vi "Setup.vi"() -> ()   [LabVIEW 2014]
uses:
  Controls/State typedef.ctl
  <vilib>/vision/NI_Vision_Development_Module.lvlib
panel:
  in  "update":bool
  out "updating":i32(slide)=250 scale=0.0..250.0
  in  "Progress...":u32(slide) min=400 max=47374 scale=0.0..21744.0
  in  "hori":cluster{i32, i32}(slide) scale=0.0..720.0
  in  "vert":cluster{i32, i32}(slide)
  out "Video play":T1(plugin-control)
  in  "START":bool
  in  "Data file":path caption="Data"
  in  "Video file":path caption="Video"
  in  "Set end":bool
  out "Start":dbl=1.0 min=0.25 max=4.0 step=0.25
  in  "Set start":bool
  out "End":dbl=1.0 min=0.25 max=4.0 step=0.25
  in  "Pause Button 2":bool
  in  "Play back\nsettings":dbl=1.0 min=0.25 max=4.0 step=0.25
  out "output array":dbl[](array[numeric])
  in  "frame jump":i32=1 min=1 max=30
  in  "Seek Forward Button":bool
  in  "Seek Back Button":bool
  in  "Pause Button":bool
  in  "Media Stop Button":bool
  in  "Play Button":bool
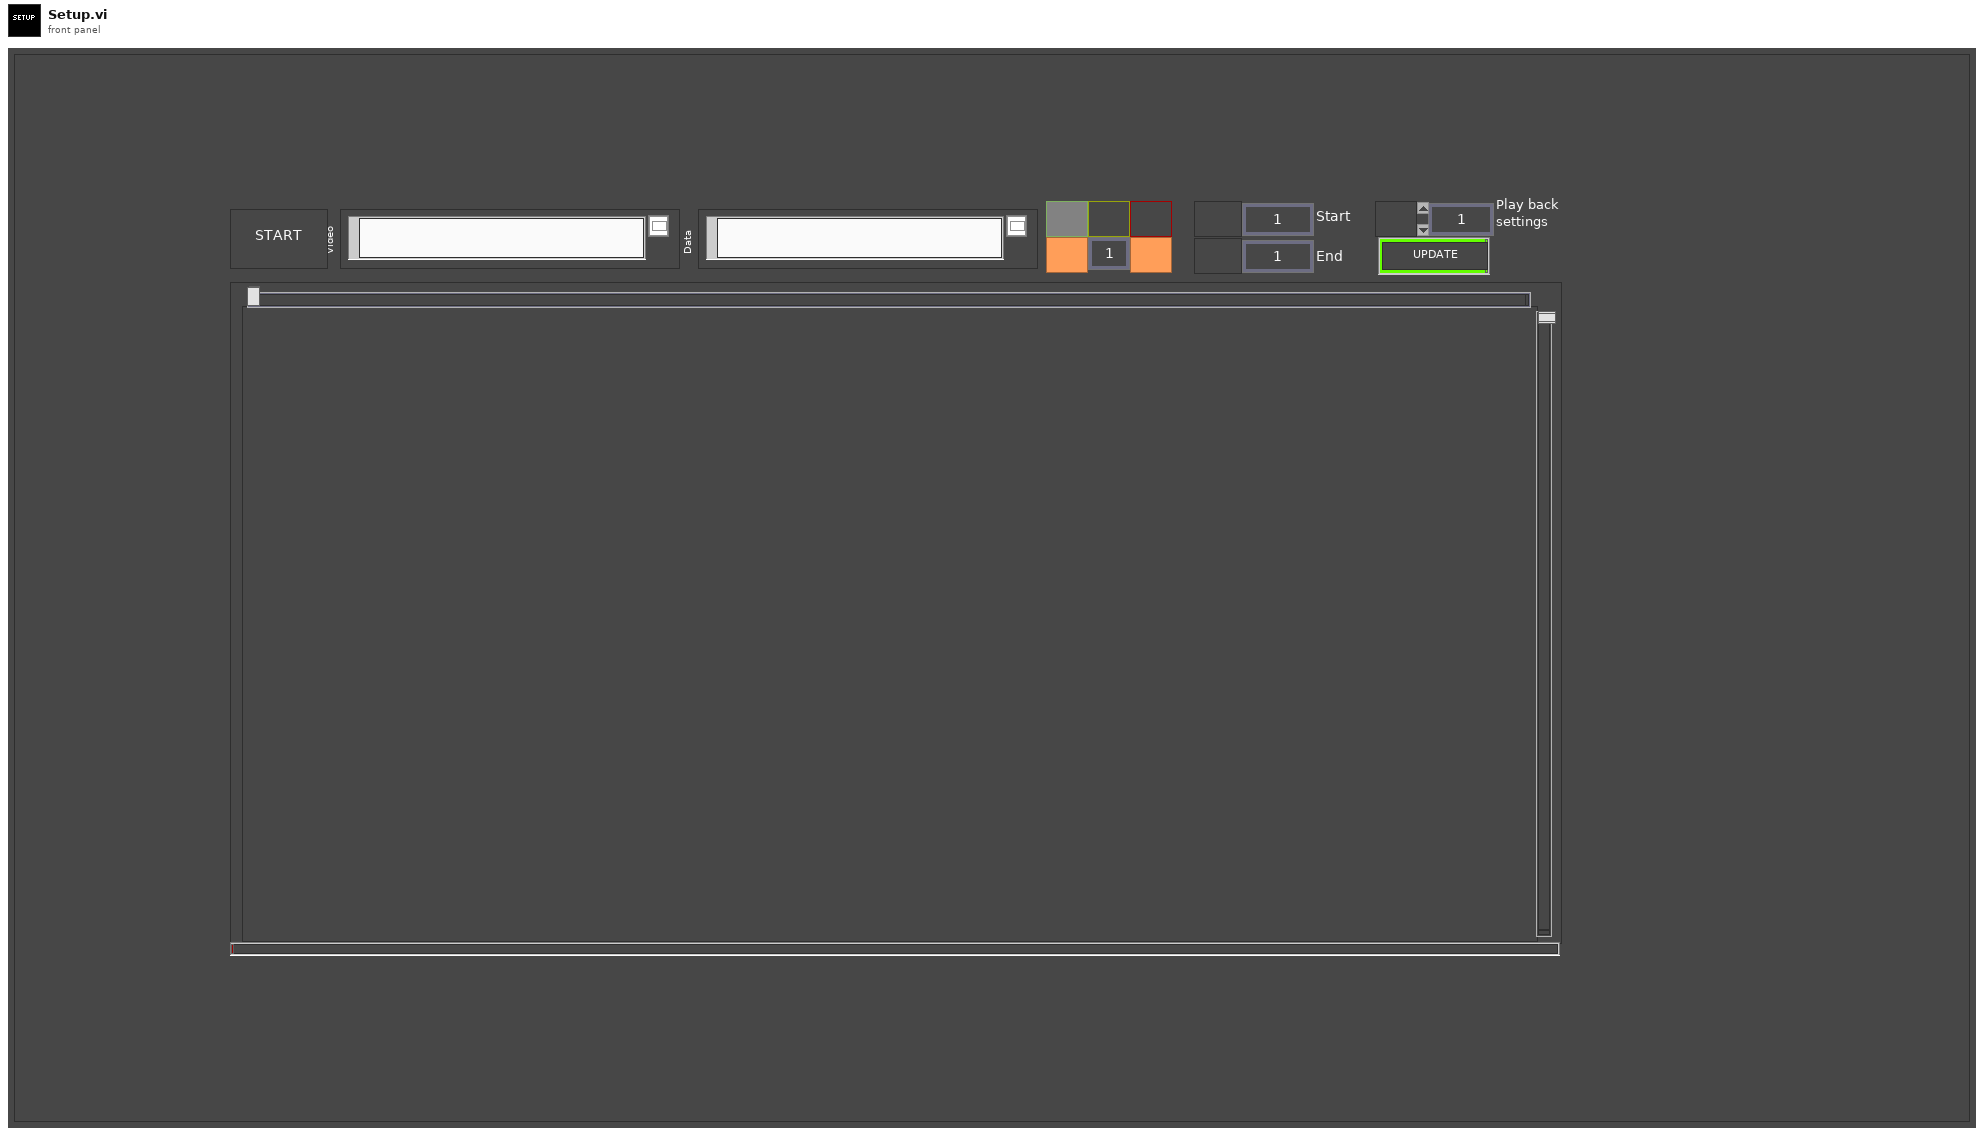
[diagram p1: front panel]
types:
  T1 = typedef "IMAQ Image.ctl" = refnum<image>
  T2 = typedef "State typedef.ctl" = enum16{"innit", "stop", "Pause", "Play", "Wait", "update"}
  T3 = typedef "Image Type" = u32
  T4 = enum16{"open", "replace", "create", "open or create", "replace or create", "replace or create with confirmation"}
  T5 = typedef "AviRefnum.ctl" = refnum<k1>
  T6 = cluster{"width":u32, "height":u32, "framesPerSecond":u32, "compressionFilter":string, "hasData":bool}
  T7 = cluster{"ID":enum32{"External", "Internal"}, "Type":u32, "Coordinates":i32[]}
  T8 = typedef "ROI Descriptor" = cluster{"Global Rectangle":i32[], "Contours":cluster{"ID":enum32{"External", "Internal"}, "Type":u32, "Coordinates":i32[]}[]}
  T9 = enum8{"Enabled", "Disabled", "Disabled and Grayed Out"}
  T10 = cluster{"ID":enum32{"External", "Internal"}, "Type":u32, "Coordinates":i32[]}[]
  T11 = typedef "eventvkey.ctl" = enum16{"ASCII", "Enter", "Return", "Shift", "Ctrl", "Alt", "Cmd", "Opt", "Caps", "NumLock", "Clear", "Break", "Up", "Down", "Left", "Right", "Insert", "Delete", "Home", "End", "PageUp", "PageDown", "Escape", "Help", "Pause", "ScrollLock", "F1", "F2", "F3", "F4", "F5", "F6", "F7", "F8", "F9", "F10", "F11", "F12", "F13", "F14", "F15", "F16", "F17", "F18", "F19", "F20", "F21", "F22", "F23", "F24", "Play", "VolumeUp", "VolumeDown", "Mute", "Two Byte Char"}
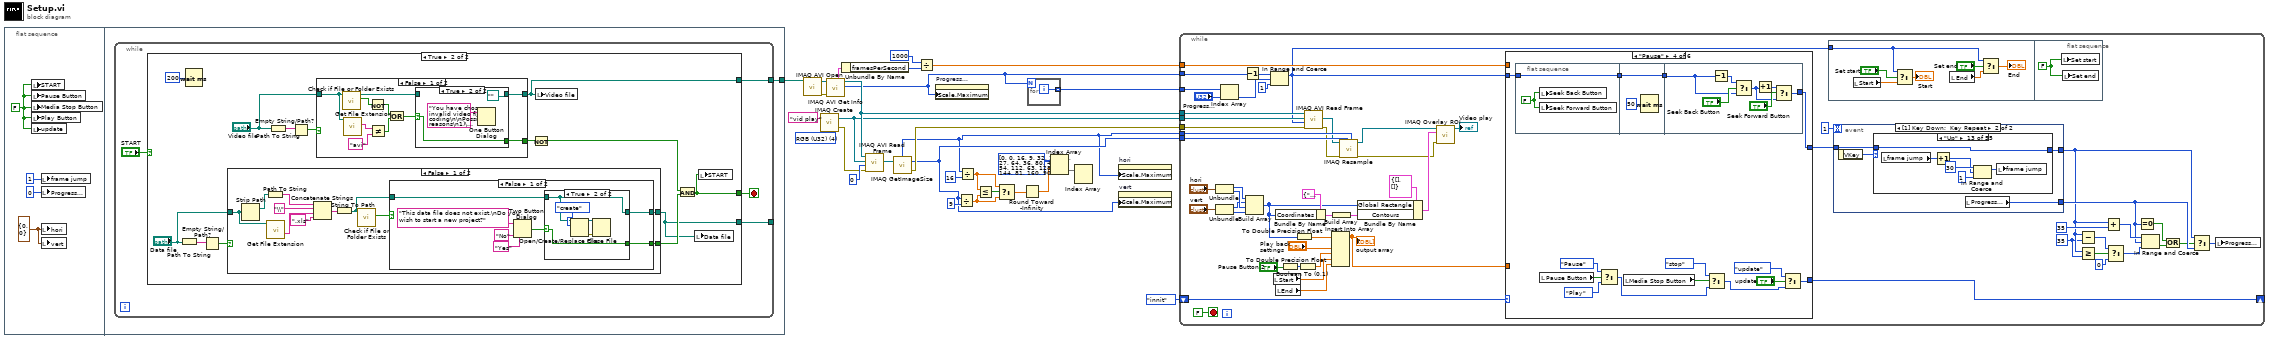
[diagram p0: block diagram]
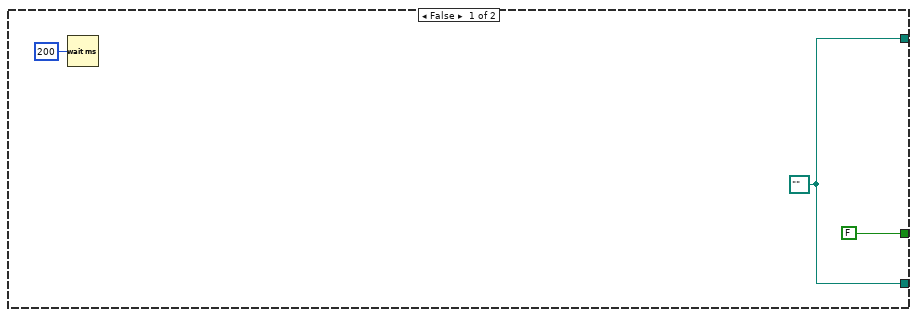
[diagram p2: hidden frame]
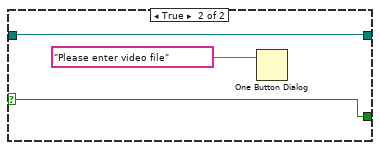
[diagram p4: hidden frame]
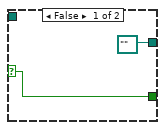
[diagram p5: hidden frame]
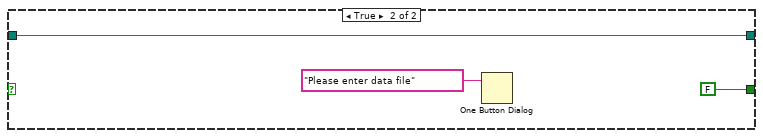
[diagram p7: hidden frame]
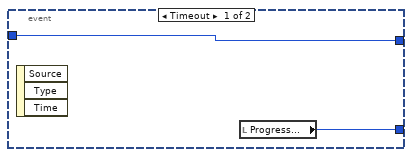
[diagram p8: hidden frame]
diagram:
  w29 = T3 4 items=["Grayscale (U8)", "Grayscale (I16)", "Grayscale (SGL)", "Complex (CSG)", "RGB (U32)", "HSL (U32)", "RGB (U64)", "Grayscale (U16)"] ("Image Type")
  n1 = flat-sequence {
    tunnel: [w34] -> w5
    frame #0 {
      w30 = cluster{i32, i32} {0, 0} ("hori")
      w31 = FALSE ("Media Stop Button")
      n2 = local write "START"(w31) -> ()
      n3 = local write "Pause Button"(w31) -> ()
      n4 = local write "Media Stop Button"(w31) -> ()
      n5 = local write "Play Button"(w31) -> ()
      n6 = local write "update"(w31) -> ()
      n7 = local write "frame jump"(1 ("frame jump")) -> ()
      n8 = local write "Progress..."(u32 0 ("Progress...")) -> ()
      n9 = local write "hori"(w30) -> ()
      n10 = local write "vert"(w30) -> ()
    }
    frame #1 {
      n11 = while {
        tunnel: [w36] -> w34
        tunnel: [w35] -> _
        stop <- w37 stop-if-true
        n12 = case shown="True" "START" {
          tunnel: [FALSE w42] -> w37
          tunnel: [w39 w45] -> w36
          tunnel: [w39 w44] -> w35
          frame False {
            w39 = path "" ("dup path")
            n13 = Wait (ms)(milliseconds to wait=u32 200) -> ()  [unwired: 1 out]
          }
          frame True {
            n14 = Path To String(path="Data file") -> (string=w54:string)
            n15 = Wait (ms)(milliseconds to wait=u32 200) -> ()  [unwired: 1 out]
            n16 = Empty String/Path?(string/path=w54) -> (empty?=w53:bool)
            n17 = case shown="False" w53 {
              tunnel: "Data file" -> [w75 w100]
              tunnel: [w74 FALSE] -> w51
              tunnel: [w73 w100] -> w44
              frame False {
                n18 = Strip Path(path=w75) -> (stripped path=w80:path)  [unwired: 1 out]
                n19 = Path To String(path=w80) -> (string=w79:string)
                n20 = call <vilib>:"Get File Extension.vi"("file"=w75) -> ("filename without extension"=w82:string)  [unwired: 7 in, 3 out]
                n21 = Concatenate Strings(w79, "\\" ("string"), w82, ".xls" ("string")) -> (w81:string)
                n22 = String To Path(string=w81) -> (path=w76:path)
                n23 = call <vilib>:"Check if File or Folder Exists.vi"("path"=w76) -> ("file or folder exists?"=w77:bool)  [unwired: 8 in, 2 out]
                n24 = case shown="False" w77 {
                  selector: w77 -> [_ w99]
                  tunnel: w76 -> [w86 w98]
                  tunnel: [w85 w99] -> w74
                  tunnel: [w84 w98] -> w73
                  frame False {
                    n25 = Two Button Dialog(message="This data file does not exist.\nDo you wish to start a new project?", 1:"No" ("F button name (\"Cancel\")"), 2:"Yes" ("T button name (\"OK\")")) -> (T button?=w87:bool)
                    n26 = case shown="True" w87 {
                      selector: w87 -> [w92 w94]
                      tunnel: w86 -> [_ w93]
                      tunnel: [w92 w94] -> w85
                      tunnel: [path "" ("dup path") w93] -> w84
                      frame False {
                      }
                      frame True {
                        n27 = Open/Create/Replace File(file path (use dialog)=w93, operation (0:open)=T4."create") -> (refnum out=w95:refnum<file>, error out=w97:errorcluster)  [unwired: 4 in, 1 out]
                        n28 = Close File(refnum=w95, error in=w97) -> ()  [unwired: 2 out]
                      }
                    }
                  }
                  frame True {
                  }
                }
              }
              frame True {
                n29 = One Button Dialog(message="Please enter data file") -> ()  [unwired: 1 in, 1 out]
              }
            }
            n30 = Path To String(path="Video file") -> (string=w49:string)
            n31 = Empty String/Path?(string/path=w49) -> (empty?=w48:bool)
            n32 = case shown="False" w48 {
              selector: w48 -> [_ w72]
              tunnel: "Video file" -> [w59 w70]
              tunnel: [w56 w70] -> w45
              tunnel: [w55 w72] -> w46
              frame False {
                n33 = call <vilib>:"Check if File or Folder Exists.vi"("path"=w59) -> ("file or folder exists?"=w63:bool, "dup path"=w57:path)  [unwired: 8 in, 1 out]
                n34 = call <vilib>:"Get File Extension.vi"("file"=w59) -> ("lowercase file extension"=w60:string)  [unwired: 7 in, 3 out]
                n35 = Not(x=w63) -> (.not. x?=w64:bool)
                n36 = Not Equal?(x=w60, y="avi" ("lowercase file extension")) -> (x != y?=w62:bool)
                n37 = Or(x=w64, y=w62) -> (x .or. y?=w58:bool)
                n38 = case shown="True" w58 {
                  selector: w58 -> [w65 w67]
                  tunnel: w57 -> [w66 _]
                  tunnel: [w66 path "" ("dup path")] -> w56
                  tunnel: [w65 w67] -> w55
                  frame False {
                  }
                  frame True {
                    n39 = One Button Dialog(message="You have chosen an invalid video file for coding\n\nPossible reasons\n1)\tChosen video file format was not AVI\n2)\tChosen video file does not exist") -> ()  [unwired: 1 in, 1 out]
                  }
                }
              }
              frame True {
                n40 = One Button Dialog(message="Please enter video file") -> ()  [unwired: 1 in, 1 out]
              }
            }
            n41 = Not(x=w46) -> (.not. x?=w50:bool)
            n42 = local write "Video file"(w45) -> ()
            n43 = And(x=w50, y=w51) -> (x .and. y?=w42:bool)
            n44 = local write "Data file"(w44) -> ()
            n45 = local write "START"(w42) -> ()
          }
        }
      }
    }
  }
  n46 = call "IMAQ AVI Open"("AVI Path"=w5) -> ("error out"=w14:errorcluster, "Avi Refnum"=w13:T5)  [unwired: 9 in]
  n47 = call "IMAQ Create"("Image Name"="vid play", "Image Type"=w29) -> ("New Image"=w11:T1, "error out"=w9:errorcluster)  [unwired: 3 in]
  n48 = call "IMAQ AVI Get Info"("error in (no error)"=w14, "Avi Refnum"=w13) -> ("Number of Frames"=w4:u32, "Avi Refnum (duplicate)"=w12:T5, "Frame Data"=w6:T6)  [unwired: 5 in, 2 out]
  n49 = Unbundle By Name(w6) -> ("framesPerSecond"=w7:u32)
  n50 = call "IMAQ AVI Read Frame"("error in (no error)"=w9, "Frame Number"=u32 0, "Image"=w11, "Avi Refnum"=w12) -> ("Image Out"=w8:T1)  [unwired: 4 in, 3 out]
  n51 = call "IMAQ GetImageSize"("Image"=w8) -> ("Y Resolution"=w2:i32, "X Resolution"=w1:i32, "error out"=w24:errorcluster)  [unwired: 3 in]
  n52 = Divide(x=1000, y=w7) -> (x/y=w25:dbl)
  n53 = property on="Progress..." class="Slide (strict)"("Scale.Maximum"=w4) -> ()  [unwired: 2 in, 2 out]
  n54 = Divide(x=w2, y=9) -> (x/y=w19:dbl)
  n55 = Divide(x=w1, y=16) -> (x/y=w20:dbl)
  n56 = Less Or Equal?(x=w20, y=w19) -> (x <= y?=w21:bool)
  n57 = Select(t=w20, s=w21, f=w19) -> (s? t:f=w17:dbl)
  n58 = Round Toward -Infinity(1:w17) -> (0:w16:dbl)
  n59 = for {
    N: w4 -> [_]
    tunnel: [w103] -> w3 mode=indexing
    i -> [w103]
  }
  n60 = Index Array(array=i32[][] [[0, 0], [16, 9], [32, 18], [48, 27], [64, 36], [80, 45], [96, 54], [112, 63], [128, 72], [144, 81], [160, 90], [176, 99], [192, 108], [208, 117], [224, 126], [240, 135], [256, 144], [272, 153], [288, 162], [304, 171], [320, 180], [336, 189], [352, 198], [368, 207], [384, 216], [400, 225], [416, 234], [432, 243], [448, 252], [464, 261], [480, 270], [496, 279], [512, 288], [528, 297], [544, 306], [560, 315], [576, 324], [592, 333], [608, 342], [624, 351], [640, 360], [656, 369], [672, 378], [688, 387], [704, 396], [720, 405], [736, 414], [752, 423], [768, 432], [784, 441], [800, 450], [816, 459], [832, 468], [848, 477], [864, 486], [880, 495], [896, 504], [912, 513], [928, 522], [944, 531], [960, 540], [976, 549], [992, 558], [1008, 567], [1024, 576], [1040, 585], [1056, 594], [1072, 603], [1088, 612], [1104, 621], [1120, 630], [1136, 639], [1152, 648], [1168, 657], [1184, 666], [1200, 675], [1216, 684], [1232, 693], [1248, 702], [1264, 711], [1280, 720], [1296, 729], [1312, 738], [1328, 747], [1344, 756], [1360, 765], [1376, 774], [1392, 783], [1408, 792], [1424, 801], [1440, 810], [1456, 819], [1472, 828], [1488, 837], [1504, 846], [1520, 855], [1536, 864], [1552, 873], [1568, 882], [1584, 891], [1600, 900], [1616, 909], [1632, 918], [1648, 927], [1664, 936], [1680, 945], [1696, 954], [1712, 963], [1728, 972], [1744, 981], [1760, 990], [1776, 999], [1792, 1008], [1808, 1017], [1824, 1026], [1840, 1035], [1856, 1044], [1872, 1053], [1888, 1062], [1904, 1071], [1920, 1080], [1936, 1089], [1952, 1098], [1968, 1107], [1984, 1116], [2000, 1125], [2016, 1134], [2032, 1143], [2048, 1152], [2064, 1161], [2080, 1170], [2096, 1179], [2112, 1188], [2128, 1197], [2144, 1206], [2160, 1215], [2176, 1224], [2192, 1233], [2208, 1242], [2224, 1251], [2240, 1260], [2256, 1269], [2272, 1278], [2288, 1287], [2304, 1296], [2320, 1305], [2336, 1314], [2352, 1323], [2368, 1332], [2384, 1341], [2400, 1350], [2416, 1359], [2432, 1368], [2448, 1377], [2464, 1386], [2480, 1395], [2496, 1404], [2512, 1413], [2528, 1422], [2544, 1431], [2560, 1440], [2576, 1449], [2592, 1458], [2608, 1467], [2624, 1476], [2640, 1485], [2656, 1494], [2672, 1503], [2688, 1512], [2704, 1521], [2720, 1530], [2736, 1539], [2752, 1548], [2768, 1557], [2784, 1566], [2800, 1575], [2816, 1584], [2832, 1593], [2848, 1602], [2864, 1611], [2880, 1620], [2896, 1629], [2912, 1638], [2928, 1647], [2944, 1656], [2960, 1665], [2976, 1674], [2992, 1683], [3008, 1692], [3024, 1701], [3040, 1710], [3056, 1719], [3072, 1728], [3088, 1737], [3104, 1746], [3120, 1755], [3136, 1764], [3152, 1773], [3168, 1782], [3184, 1791], [3200, 1800], [3216, 1809], [3232, 1818], [3248, 1827], [3264, 1836], [3280, 1845], [3296, 1854], [3312, 1863], [3328, 1872], [3344, 1881], [3360, 1890], [3376, 1899], [3392, 1908], [3408, 1917], [3424, 1926], [3440, 1935], [3456, 1944], [3472, 1953], [3488, 1962], [3504, 1971], [3520, 1980], [3536, 1989], [3552, 1998], [3568, 2007], [3584, 2016], [3600, 2025], [3616, 2034], [3632, 2043], [3648, 2052], [3664, 2061], [3680, 2070], [3696, 2079], [3712, 2088], [3728, 2097], [3744, 2106], [3760, 2115], [3776, 2124], [3792, 2133], [3808, 2142], [3824, 2151], [3840, 2160], [3856, 2169], [3872, 2178], [3888, 2187], [3904, 2196], [3920, 2205], [3936, 2214], [3952, 2223], [3968, 2232], [3984, 2241], [4000, 2250], [4016, 2259], [4032, 2268], [4048, 2277], [4064, 2286], [4080, 2295], [4096, 2304], [4112, 2313], [4128, 2322], [4144, 2331], [4160, 2340], [4176, 2349], [4192, 2358], [4208, 2367], [4224, 2376], [4240, 2385], [4256, 2394], [4272, 2403], [4288, 2412], [4304, 2421], [4320, 2430], [4336, 2439], [4352, 2448], [4368, 2457], [4384, 2466], [4400, 2475], [4416, 2484], [4432, 2493], [4448, 2502], [4464, 2511], [4480, 2520], [4496, 2529], [4512, 2538], [4528, 2547], [4544, 2556], [4560, 2565], [4576, 2574], [4592, 2583], [4608, 2592], [4624, 2601], [4640, 2610], [4656, 2619], [4672, 2628], [4688, 2637], [4704, 2646], [4720, 2655], [4736, 2664], [4752, 2673], [4768, 2682], [4784, 2691], [4800, 2700], [4816, 2709], [4832, 2718], [4848, 2727], [4864, 2736], [4880, 2745], [4896, 2754], [4912, 2763], [4928, 2772], [4944, 2781], [4960, 2790], [4976, 2799], [4992, 2808], [5008, 2817], [5024, 2826], [5040, 2835], [5056, 2844], [5072, 2853], [5088, 2862], [5104, 2871], [5120, 2880], [5136, 2889], [5152, 2898], [5168, 2907], [5184, 2916], [5200, 2925], [5216, 2934], [5232, 2943], [5248, 2952], [5264, 2961], [5280, 2970], [5296, 2979], [5312, 2988], [5328, 2997], [5344, 3006], [5360, 3015], [5376, 3024], [5392, 3033], [5408, 3042], [5424, 3051], [5440, 3060], [5456, 3069], [5472, 3078], [5488, 3087], [5504, 3096], [5520, 3105], [5536, 3114], [5552, 3123], [5568, 3132], [5584, 3141], [5600, 3150], [5616, 3159], [5632, 3168], [5648, 3177], [5664, 3186], [5680, 3195], [5696, 3204], [5712, 3213], [5728, 3222], [5744, 3231], [5760, 3240], [5776, 3249], [5792, 3258], [5808, 3267], [5824, 3276], [5840, 3285], [5856, 3294], [5872, 3303], [5888, 3312], [5904, 3321], [5920, 3330], [5936, 3339], [5952, 3348], [5968, 3357], [5984, 3366], [6000, 3375], [6016, 3384], [6032, 3393], [6048, 3402], [6064, 3411], [6080, 3420], [6096, 3429], [6112, 3438], [6128, 3447], [6144, 3456], [6160, 3465], [6176, 3474], [6192, 3483], [6208, 3492], [6224, 3501], [6240, 3510], [6256, 3519], [6272, 3528], [6288, 3537], [6304, 3546], [6320, 3555], [6336, 3564], [6352, 3573], [6368, 3582], [6384, 3591], [6400, 3600], [6416, 3609], [6432, 3618], [6448, 3627], [6464, 3636], [6480, 3645], [6496, 3654], [6512, 3663], [6528, 3672], [6544, 3681], [6560, 3690], [6576, 3699], [6592, 3708], [6608, 3717], [6624, 3726], [6640, 3735], [6656, 3744], [6672, 3753], [6688, 3762], [6704, 3771], [6720, 3780], [6736, 3789], [6752, 3798], [6768, 3807], [6784, 3816], [6800, 3825], [6816, 3834], [6832, 3843], [6848, 3852], [6864, 3861], [6880, 3870], [6896, 3879], [6912, 3888], [6928, 3897], [6944, 3906], [6960, 3915], [6976, 3924], [6992, 3933], [7008, 3942], [7024, 3951], [7040, 3960], [7056, 3969], [7072, 3978], [7088, 3987], [7104, 3996], [7120, 4005], [7136, 4014], [7152, 4023], [7168, 4032], [7184, 4041], [7200, 4050], [7216, 4059], [7232, 4068], [7248, 4077], [7264, 4086], [7280, 4095], [7296, 4104], [7312, 4113], [7328, 4122], [7344, 4131], [7360, 4140], [7376, 4149], [7392, 4158], [7408, 4167], [7424, 4176], [7440, 4185], [7456, 4194], [7472, 4203], [7488, 4212], [7504, 4221], [7520, 4230], [7536, 4239], [7552, 4248], [7568, 4257], [7584, 4266], [7600, 4275], [7616, 4284], [7632, 4293], [7648, 4302], [7664, 4311], [7680, 4320], [7696, 4329], [7712, 4338], [7728, 4347], [7744, 4356], [7760, 4365], [7776, 4374], [7792, 4383], [7808, 4392], [7824, 4401], [7840, 4410], [7856, 4419], [7872, 4428], [7888, 4437], [7904, 4446], [7920, 4455], [7936, 4464], [7952, 4473], [7968, 4482], [7984, 4491], [8000, 4500], [8016, 4509], [8032, 4518], [8048, 4527], [8064, 4536], [8080, 4545], [8096, 4554], [8112, 4563], [8128, 4572], [8144, 4581], [8160, 4590], [8176, 4599], [8192, 4608], [8208, 4617], [8224, 4626], [8240, 4635], [8256, 4644], [8272, 4653], [8288, 4662], [8304, 4671], [8320, 4680], [8336, 4689], [8352, 4698], [8368, 4707], [8384, 4716], [8400, 4725], [8416, 4734], [8432, 4743], [8448, 4752], [8464, 4761], [8480, 4770], [8496, 4779], [8512, 4788], [8528, 4797], [8544, 4806], [8560, 4815], [8576, 4824], [8592, 4833], [8608, 4842], [8624, 4851], [8640, 4860], [8656, 4869], [8672, 4878], [8688, 4887], [8704, 4896], [8720, 4905], [8736, 4914], [8752, 4923], [8768, 4932], [8784, 4941], [8800, 4950], [8816, 4959], [8832, 4968], [8848, 4977], [8864, 4986], [8880, 4995], [8896, 5004], [8912, 5013], [8928, 5022], [8944, 5031], [8960, 5040], [8976, 5049], [8992, 5058], [9008, 5067], [9024, 5076], [9040, 5085], [9056, 5094], [9072, 5103], [9088, 5112], [9104, 5121], [9120, 5130], [9136, 5139], [9152, 5148], [9168, 5157], [9184, 5166], [9200, 5175], [9216, 5184], [9232, 5193], [9248, 5202], [9264, 5211], [9280, 5220], [9296, 5229], [9312, 5238], [9328, 5247], [9344, 5256], [9360, 5265], [9376, 5274], [9392, 5283], [9408, 5292], [9424, 5301], [9440, 5310], [9456, 5319], [9472, 5328], [9488, 5337], [9504, 5346], [9520, 5355], [9536, 5364], [9552, 5373], [9568, 5382], [9584, 5391], [9600, 5400], [9616, 5409], [9632, 5418], [9648, 5427], [9664, 5436], [9680, 5445], [9696, 5454], [9712, 5463], [9728, 5472], [9744, 5481], [9760, 5490], [9776, 5499], [9792, 5508], [9808, 5517], [9824, 5526], [9840, 5535], [9856, 5544], [9872, 5553], [9888, 5562], [9904, 5571], [9920, 5580], [9936, 5589], [9952, 5598], [9968, 5607], [9984, 5616], [10000, 5625], [10016, 5634], [10032, 5643], [10048, 5652], [10064, 5661], [10080, 5670], [10096, 5679], [10112, 5688], [10128, 5697], [10144, 5706], [10160, 5715], [10176, 5724], [10192, 5733], [10208, 5742], [10224, 5751], [10240, 5760], [10256, 5769], [10272, 5778], [10288, 5787], [10304, 5796], [10320, 5805], [10336, 5814], [10352, 5823], [10368, 5832], [10384, 5841], [10400, 5850], [10416, 5859], [10432, 5868], [10448, 5877], [10464, 5886], [10480, 5895], [10496, 5904], [10512, 5913], [10528, 5922], [10544, 5931], [10560, 5940], [10576, 5949], [10592, 5958], [10608, 5967], [10624, 5976], [10640, 5985], [10656, 5994], [10672, 6003], [10688, 6012], [10704, 6021], [10720, 6030], [10736, 6039], [10752, 6048], [10768, 6057], [10784, 6066], [10800, 6075], [10816, 6084], [10832, 6093], [10848, 6102], [10864, 6111], [10880, 6120], [10896, 6129], [10912, 6138], [10928, 6147], [10944, 6156], [10960, 6165], [10976, 6174], [10992, 6183], [11008, 6192], [11024, 6201], [11040, 6210], [11056, 6219], [11072, 6228], [11088, 6237], [11104, 6246], [11120, 6255], [11136, 6264], [11152, 6273], [11168, 6282], [11184, 6291], [11200, 6300], [11216, 6309], [11232, 6318], [11248, 6327], [11264, 6336], [11280, 6345], [11296, 6354], [11312, 6363], [11328, 6372], [11344, 6381], [11360, 6390], [11376, 6399], [11392, 6408], [11408, 6417], [11424, 6426], [11440, 6435], [11456, 6444], [11472, 6453], [11488, 6462], [11504, 6471], [11520, 6480], [11536, 6489], [11552, 6498], [11568, 6507], [11584, 6516], [11600, 6525], [11616, 6534], [11632, 6543], [11648, 6552], [11664, 6561], [11680, 6570], [11696, 6579], [11712, 6588], [11728, 6597], [11744, 6606], [11760, 6615], [11776, 6624], [11792, 6633], [11808, 6642], [11824, 6651], [11840, 6660], [11856, 6669], [11872, 6678], [11888, 6687], [11904, 6696], [11920, 6705], [11936, 6714], [11952, 6723], [11968, 6732], [11984, 6741], [12000, 6750], [12016, 6759], [12032, 6768], [12048, 6777], [12064, 6786], [12080, 6795], [12096, 6804], [12112, 6813], [12128, 6822], [12144, 6831], [12160, 6840], [12176, 6849], [12192, 6858], [12208, 6867], [12224, 6876], [12240, 6885], [12256, 6894], [12272, 6903], [12288, 6912], [12304, 6921], [12320, 6930], [12336, 6939], [12352, 6948], [12368, 6957], [12384, 6966], [12400, 6975], [12416, 6984], [12432, 6993], [12448, 7002], [12464, 7011], [12480, 7020], [12496, 7029], [12512, 7038], [12528, 7047], [12544, 7056], [12560, 7065], [12576, 7074], [12592, 7083], [12608, 7092], [12624, 7101], [12640, 7110], [12656, 7119], [12672, 7128], [12688, 7137], [12704, 7146], [12720, 7155], [12736, 7164], [12752, 7173], [12768, 7182], [12784, 7191], [12800, 7200], [12816, 7209], [12832, 7218], [12848, 7227], [12864, 7236], [12880, 7245], [12896, 7254], [12912, 7263], [12928, 7272], [12944, 7281], [12960, 7290], [12976, 7299], [12992, 7308], [13008, 7317], [13024, 7326], [13040, 7335], [13056, 7344], [13072, 7353], [13088, 7362], [13104, 7371], [13120, 7380], [13136, 7389], [13152, 7398], [13168, 7407], [13184, 7416], [13200, 7425], [13216, 7434], [13232, 7443], [13248, 7452], [13264, 7461], [13280, 7470], [13296, 7479], [13312, 7488], [13328, 7497], [13344, 7506], [13360, 7515], [13376, 7524], [13392, 7533], [13408, 7542], [13424, 7551], [13440, 7560], [13456, 7569], [13472, 7578], [13488, 7587], [13504, 7596], [13520, 7605], [13536, 7614], [13552, 7623], [13568, 7632], [13584, 7641], [13600, 7650], [13616, 7659], [13632, 7668], [13648, 7677], [13664, 7686], [13680, 7695], [13696, 7704], [13712, 7713], [13728, 7722], [13744, 7731], [13760, 7740], [13776, 7749], [13792, 7758], [13808, 7767], [13824, 7776], [13840, 7785], [13856, 7794], [13872, 7803], [13888, 7812], [13904, 7821], [13920, 7830], [13936, 7839], [13952, 7848], [13968, 7857], [13984, 7866], [14000, 7875], [14016, 7884], [14032, 7893], [14048, 7902], [14064, 7911], [14080, 7920], [14096, 7929], [14112, 7938], [14128, 7947], [14144, 7956], [14160, 7965], [14176, 7974], [14192, 7983], [14208, 7992], [14224, 8001], [14240, 8010], [14256, 8019], [14272, 8028], [14288, 8037], [14304, 8046], [14320, 8055], [14336, 8064], [14352, 8073], [14368, 8082], [14384, 8091], [14400, 8100], [14416, 8109], [14432, 8118], [14448, 8127], [14464, 8136], [14480, 8145], [14496, 8154], [14512, 8163], [14528, 8172], [14544, 8181], [14560, 8190], [14576, 8199], [14592, 8208], [14608, 8217], [14624, 8226], [14640, 8235], [14656, 8244], [14672, 8253], [14688, 8262], [14704, 8271], [14720, 8280], [14736, 8289], [14752, 8298], [14768, 8307], [14784, 8316], [14800, 8325], [14816, 8334], [14832, 8343], [14848, 8352], [14864, 8361], [14880, 8370], [14896, 8379], [14912, 8388], [14928, 8397], [14944, 8406], [14960, 8415], [14976, 8424], [14992, 8433], [15008, 8442], [15024, 8451], [15040, 8460], [15056, 8469], [15072, 8478], [15088, 8487], [15104, 8496], [15120, 8505], [15136, 8514], [15152, 8523], [15168, 8532], [15184, 8541], [15200, 8550], [15216, 8559], [15232, 8568], [15248, 8577], [15264, 8586], [15280, 8595], [15296, 8604], [15312, 8613], [15328, 8622], [15344, 8631], [15360, 8640], [15376, 8649], [15392, 8658], [15408, 8667], [15424, 8676], [15440, 8685], [15456, 8694], [15472, 8703], [15488, 8712], [15504, 8721], [15520, 8730], [15536, 8739], [15552, 8748], [15568, 8757], [15584, 8766], [15600, 8775], [15616, 8784], [15632, 8793], [15648, 8802], [15664, 8811], [15680, 8820], [15696, 8829], [15712, 8838], [15728, 8847], [15744, 8856], [15760, 8865], [15776, 8874], [15792, 8883], [15808, 8892], [15824, 8901], [15840, 8910], [15856, 8919], [15872, 8928], [15888, 8937], [15904, 8946], [15920, 8955], [15936, 8964], [15952, 8973], [15968, 8982], [15984, 8991]] ("appended array"), index (row)=w16) -> (element=w15:i32[])  [unwired: 1 in]
  n61 = Index Array(array=w15) -> ()  [unwired: 2 in, 2 out]
  n62 = property on="hori" class="Slide (strict)"("Scale.Maximum"=w1) -> ()  [unwired: 2 in, 2 out]
  n63 = property on="vert" class="Slide (strict)"("Scale.Maximum"=w2) -> ()  [unwired: 2 in, 2 out]
  n64 = while {
    tunnel: w24 -> [w147]
    tunnel: w12 -> [w148]
    tunnel: w11 -> [w146]
    shift-right: [w157] -> _
    shift-left: State_typedef."innit" ("Enum") -> [w159]
    tunnel: w4 -> [w155]
    tunnel: w25 -> [w125]
    tunnel: w1 -> [w151]
    tunnel: w2 -> [w150]
    tunnel: w3 -> [w122]
    stop <- FALSE stop-if-true
    w108 = u32 35 ("y")
    n65 = Unbundle("hori") -> (w139:i32, w141:i32)
    n66 = Unbundle("vert") -> (w140:i32, w142:i32)
    n67 = Index Array(array=w122, index="Progress...") -> (element=w120:i32)
    n68 = Decrement(x=w155) -> (x-1=w156:u32)
    n69 = Build Array(w139, w140, w141, w142) -> (w130:i32[])
    n70 = In Range and Coerce(upper limit=w156, x=w120, lower limit=u32 1) -> (coerced(x)=w119:u32)  [unwired: 1 out]
    n71 = local read "Start"() -> (w124:dbl)
    n72 = Bundle By Name(cluster=T7 {"ID"=enum."External", "Type"=3, "Coordinates"=[]}, "Coordinates"=w130) -> (w143:T7)
    n73 = local read "End"() -> (w123:dbl)
    n74 = Boolean To (0,1)(Boolean="Pause Button 2") -> (0, 1=w128:i16)
    n75 = To Double Precision Float(number=w130) -> (double precision float=w129:dbl[])
    n76 = To Double Precision Float(number=w128) -> (double precision float=w127:dbl)
    n77 = call "IMAQ AVI Read Frame"("error in (no error)"=w147, "Frame Number"=w119, "Image"=w146, "Avi Refnum"=w148) -> ("error out"=w132:errorcluster, "Image Out"=w145:T1)  [unwired: 4 in, 2 out]
    n78 = Insert Into Array(array=w129, new element #1="Play back\nsettings", new element #2=w127, new element #3=w124, new element #4=w123) -> (w104:dbl[])  [unwired: 1 in]
    "output array" <- w104
    n79 = Build Array(w143) -> (w144:T10)
    n80 = call "IMAQ Resample"("X Resolution"=w151, "Y Resolution"=w150, "error in (no error)"=w132, "Image Src"=w145) -> ("error out"=w133:errorcluster, "Image Dst Out"=w149:T1)  [unwired: 6 in]
    n81 = Bundle By Name(cluster=T8 {"Global Rectangle"=[], "Contours"=[]} ("ROI Descriptor"), "Global Rectangle"=w130, "Contours"=w144) -> (w134:T8)
    n82 = call "IMAQ Overlay ROI"("error in (no error)"=w133, "ROI Descriptor"=w134, "Image"=w149) -> ("Image Out"=→"Video play":T1)  [unwired: 7 in, 1 out]
    n83 = case shown="\"Pause\"" w159 {
      tunnel: [State_typedef."Wait" ("Enum") w257 w267 w273 State_typedef."innit" ("Enum") State_typedef."Pause" ("Enum")] -> w157
      tunnel: w119 -> [w247 w251 w258 w279 _ w304]
      tunnel: [w247 w251 w262 w280 w298 w304] -> w118
      tunnel: w125 -> [_ _ w259 _ _ _]
      tunnel: w104 -> [_ _ _ _ _ w307]
      frame "innit", Default {
        w248 = T9."Disabled and Grayed Out" ("Disabled")
        w244 = FALSE ("Media Stop Button")
        n84 = property on="Pause Button" class="Bool (strict)"("DisabledEnum"=w248) -> ()  [unwired: 2 in, 2 out]
        n85 = property on="Play Button" class="Bool (strict)"("DisabledEnum"=T9."Enabled" ("Disabled")) -> ()  [unwired: 2 in, 2 out]
        n86 = local write "frame jump"(1 ("frame jump")) -> ()
        n87 = local write "Progress..."(u32 0 ("Progress...")) -> ()
        n88 = local write "Pause Button"(w244) -> ()
        n89 = local write "Media Stop Button"(w244) -> ()
        n90 = local write "Play Button"(w244) -> ()
        n91 = local write "update"(w244) -> ()
        n92 = property on="Media Stop Button" class="Bool (strict)"("DisabledEnum"=w248) -> ()  [unwired: 2 in, 2 out]
      }
      frame "Wait" {
        w252 = T9."Disabled and Grayed Out" ("Disabled")
        n93 = property on="Pause Button" class="Bool (strict)"("DisabledEnum"=w252) -> ()  [unwired: 2 in, 2 out]
        n94 = property on="Play Button" class="Bool (strict)"("DisabledEnum"=T9."Enabled" ("Disabled")) -> ()  [unwired: 2 in, 2 out]
        n95 = property on="Media Stop Button" class="Bool (strict)"("DisabledEnum"=w252) -> ()  [unwired: 2 in, 2 out]
        n96 = Select(t=State_typedef."Play" ("Enum"), s="Play Button", f=State_typedef."Wait" ("Enum")) -> (s? t:f=w257:T2)
      }
      frame "Play" {
        w260 = T9."Enabled" ("Disabled")
        n97 = Wait (ms)(milliseconds to wait=w259) -> ()  [unwired: 1 out]
        n98 = Select(t=State_typedef."Pause" ("Enum"), s="Pause Button", f=State_typedef."Play" ("Enum")) -> (s? t:f=w268:T2)
        n99 = local read "Play Button"() -> (w266:bool)
        n100 = property on="Media Stop Button" class="Bool (strict)"("DisabledEnum"=w260) -> ()  [unwired: 2 in, 2 out]
        n101 = property on="Pause Button" class="Bool (strict)"("DisabledEnum"=w260) -> ()  [unwired: 2 in, 2 out]
        n102 = property on="Play Button" class="Bool (strict)"("DisabledEnum"=T9."Disabled and Grayed Out" ("Disabled")) -> ()  [unwired: 2 in, 2 out]
        n103 = Not(x=w266) -> (.not. x?=w265:bool)
        n104 = Increment(x=w258) -> (x+1=w262:u32)
        n105 = Or(x=w265, y="Media Stop Button") -> (x .or. y?=w263:bool)
        n106 = Select(t=State_typedef."stop" ("Enum"), s=w263, f=w268) -> (s? t:f=w267:T2)
      }
      frame "Pause" {
        n107 = flat-sequence {
          tunnel: w279 -> [w287]
          tunnel: [w287] -> w277
          tunnel: [w290] -> w278
          tunnel: w277 -> [w290]
          tunnel: [w292] -> w280
          tunnel: w278 -> [w291]
          frame #0 {
            w288 = FALSE ("Seek Forward Button")
            n108 = local write "Seek Back Button"(w288) -> ()
            n109 = local write "Seek Forward Button"(w288) -> ()
          }
          frame #1 {
            n110 = Wait (ms)(milliseconds to wait=u32 50) -> ()  [unwired: 1 out]
          }
          frame #2 {
            n111 = Decrement(x=w291) -> (x-1=w295:u32)
            n112 = Select(t=w295, s="Seek Back Button", f=w291) -> (s? t:f=w293:u32)
            n113 = Increment(x=w293) -> (x+1=w296:u32)
            n114 = Select(t=w296, s="Seek Forward Button", f=w293) -> (s? t:f=w292:u32)
          }
        }
        n115 = local read "Pause Button"() -> (w286:bool)
        n116 = Select(t=State_typedef."Pause" ("Enum"), s=w286, f=State_typedef."Play" ("Enum")) -> (s? t:f=w281:T2)
        n117 = local read "Media Stop Button"() -> (w283:bool)
        n118 = Select(t=State_typedef."stop" ("Enum"), s=w283, f=w281) -> (s? t:f=w274:T2)
        n119 = Select(t=State_typedef."update" ("Enum"), s="update", f=w274) -> (s? t:f=w273:T2)
      }
      frame "stop" {
        w299 = T9."Disabled and Grayed Out" ("Disabled")
        w298 = u32 0 ("milliseconds to wait")
        w301 = FALSE ("Play Button")
        n120 = local write "Play Button"(w301) -> ()
        n121 = local write "Pause Button"(w301) -> ()
        n122 = local write "Media Stop Button"(w301) -> ()
        n123 = property on="Pause Button" class="Bool (strict)"("DisabledEnum"=w299) -> ()  [unwired: 2 in, 2 out]
        n124 = property on="Play Button" class="Bool (strict)"("DisabledEnum"=T9."Enabled" ("Disabled")) -> ()  [unwired: 2 in, 2 out]
        n125 = property on="Media Stop Button" class="Bool (strict)"("DisabledEnum"=w299) -> ()  [unwired: 2 in, 2 out]
        n126 = local write "Progress..."(w298) -> ()
      }
      frame "update" {
        n127 = Array To Spreadsheet String(array=w307, 3:"%f" ("format string")) -> (spreadsheet string=w305:string)  [unwired: 1 in]
        n128 = flat-sequence {
          tunnel: w305 -> [w313]
          frame #0 {
            n129 = local read "Data file"() -> (w315:path)
            n130 = Open/Create/Replace File(file path (use dialog)=w315, operation (0:open)=T4."open") -> (refnum out=w310:refnum<file>, error out=w311:errorcluster)  [unwired: 4 in, 1 out]
            n131 = for {
              N: 501 -> [_]
              i -> [w318]
              n132 = Wait (ms)(milliseconds to wait=u32 1) -> ()  [unwired: 1 out]
              "updating" <- w318
            }
            n133 = Read from Text File(file (use dialog)=w310, error in=w311) -> (refnum out=w309:refnum<file>, error out=w308:errorcluster)  [unwired: 2 in, 2 out]
            n134 = Write to Text File(file (use dialog)=w309, text=w313, error in=w308) -> (refnum out=w317:refnum<file>, error out=w316:errorcluster)  [unwired: 1 in, 1 out]
            n135 = Close File(refnum=w317, error in=w316) -> ()  [unwired: 2 out]
          }
          frame #1 {
            n136 = local write "update"(FALSE ("update")) -> ()
          }
        }
      }
    }
    n137 = flat-sequence {
      tunnel: w119 -> [w160]
      frame #0 {
        n138 = local read "Start"() -> (w165:dbl)
        n139 = Select(t=w160, s="Set start", f=w165) -> (s? t:f=→"Start":dbl)
        n140 = local read "End"() -> (w162:dbl)
        n141 = Select(t=w160, s="Set end", f=w162) -> (s? t:f=→"End":dbl)
      }
      frame #1 {
        w167 = FALSE ("Set end")
        n142 = local write "Set start"(w167) -> ()
        n143 = local write "Set end"(w167) -> ()
      }
    }
    n144 = event shown="[1] Key Down;  Key Repeat" {
      selector: _ -> [_ _]
      dyn-events: _ -> [_ _]
      timeout: 1 -> [_ _]
      tunnel: w118 -> [w169 w172]
      tunnel: [w169 w171] -> w109
      tunnel: [w168 w170] -> w114
      event Timeout {
        n145 = event-data() -> ()  [unwired: 1 in, 3 out]
        n146 = local read "Progress..."() -> (w168:u32)
      }
      event Key Down; Key Repeat {
        n147 = event-data() -> ("VKey"=w173:T11)  [unwired: 1 in]
        n148 = case shown="\"Up\"" w173 {
          tunnel: w172 -> [w174 w175 w176 w177 w178 w179 w180 w181 w182 w183 w184 w185 w191 w197 w201 w202 w205 w206 w207 w208 w209 w210 w211 w212 w213 w214 w215 w216 w217 w218 w219 w220 w221 w222 w223 w224 w225 w226 w227 w228 w229 w230 w231 w232 w233 w234 w235 w236 w237 w238 w239 w240 w241 w242 w243]
          tunnel: [w174 w175 w176 w177 w178 w179 w180 w181 w182 w183 w184 w185 w191 w197 w198 w204 w205 w206 w207 w208 w209 w210 w211 w212 w213 w214 w215 w216 w217 w218 w219 w220 w221 w222 w223 w224 w225 w226 w227 w228 w229 w230 w231 w232 w233 w234 w235 w236 w237 w238 w239 w240 w241 w242 w243] -> w171
          frame "ASCII", Default {
          }
          frame "Enter" {
          }
          frame "Return" {
          }
          frame "Shift" {
          }
          frame "Ctrl" {
          }
          frame "Alt" {
          }
          frame "Cmd" {
          }
          frame "Opt" {
          }
          frame "Caps" {
          }
          frame "NumLock" {
          }
          frame "Clear" {
          }
          frame "Break" {
          }
          frame "Up" {
            n149 = local read "frame jump"() -> (w190:i32)
            n150 = Increment(x=w190) -> (x+1=w187:i32)
            n151 = In Range and Coerce(upper limit=30, x=w187, lower limit=1 ("frame jump")) -> (coerced(x)=w186:i32)  [unwired: 1 out]
            n152 = local write "frame jump"(w186) -> ()
          }
          frame "Down" {
            n153 = local read "frame jump"() -> (w196:i32)
            n154 = Decrement(x=w196) -> (x-1=w193:i32)
            n155 = In Range and Coerce(upper limit=30, x=w193, lower limit=1 ("frame jump")) -> (coerced(x)=w192:i32)  [unwired: 1 out]
            n156 = local write "frame jump"(w192) -> ()
          }
          frame "Left" {
            n157 = Subtract(x=w201, y="frame jump") -> (x-y=w199:u32)
            n158 = Decrement(x=w199) -> (x-1=w198:u32)
          }
          frame "Right" {
            n159 = local read "frame jump"() -> (w203:i32)
            n160 = Add(x=w202, y=w203) -> (x+y=w204:u32)
          }
          frame "Insert" {
          }
          frame "Delete" {
          }
          frame "Home" {
          }
          frame "End" {
          }
          frame "PageUp" {
          }
          frame "PageDown" {
          }
          frame "Escape" {
          }
          frame "Help" {
          }
          frame "Pause" {
          }
          frame "ScrollLock" {
          }
          frame "F1" {
          }
          frame "F2" {
          }
          frame "F3" {
          }
          frame "F4" {
          }
          frame "F5" {
          }
          frame "F6" {
          }
          frame "F7" {
          }
          frame "F8" {
          }
          frame "F9" {
          }
          frame "F10" {
          }
          frame "F11" {
          }
          frame "F12" {
          }
          frame "F13" {
          }
          frame "F14" {
          }
          frame "F15" {
          }
          frame "F16" {
          }
          frame "F17" {
          }
          frame "F18" {
          }
          frame "F19" {
          }
          frame "F20" {
          }
          frame "F21" {
          }
          frame "F22" {
          }
          frame "F23" {
          }
          frame "F24" {
          }
          frame "Play" {
          }
          frame "VolumeUp" {
          }
          frame "VolumeDown" {
          }
          frame "Mute" {
          }
          frame "Two Byte Char" {
          }
        }
        n161 = local read "Progress..."() -> (w170:u32)
      }
    }
    n162 = Subtract(x=w109, y=w108) -> (x-y=w107:u32)
    n163 = Greater Or Equal?(x=w109, y=w108) -> (x >= y?=w110:bool)
    n164 = Add(x=w109, y=u32 35) -> (x+y=w116:u32)
    n165 = Select(t=w107, s=w110, f=u32 0) -> (s? t:f=w105:u32)
    n166 = Equal To 0?(x=w114) -> (x = 0?=w112:bool)
    n167 = In Range and Coerce(upper limit=w116, x=w114, lower limit=w105) -> (In Range?=w113:bool)  [unwired: 1 out]
    n168 = Or(x=w112, y=w113) -> (x .or. y?=w111:bool)
    n169 = Select(t=w109, s=w111, f=w114) -> (s? t:f=w115:u32)
    n170 = local write "Progress..."(w115) -> ()
  }
